vi "报文解析子VI.vi"(11 "剔除报文标识字符串":string) -> (0 "当时日期":string, 1 "速度及航向":string, 2 "经度":string, 3 "纬度":string, 4 "UTCtime":string)   [LabVIEW 2018]
panel:
  out "对地真航向":string
  out "对地速度":string
  out "ULon":string
  out "LON":string
  out "ULat":string
  out "LAT":string
  out "STATUS":u8[](array[numeric])
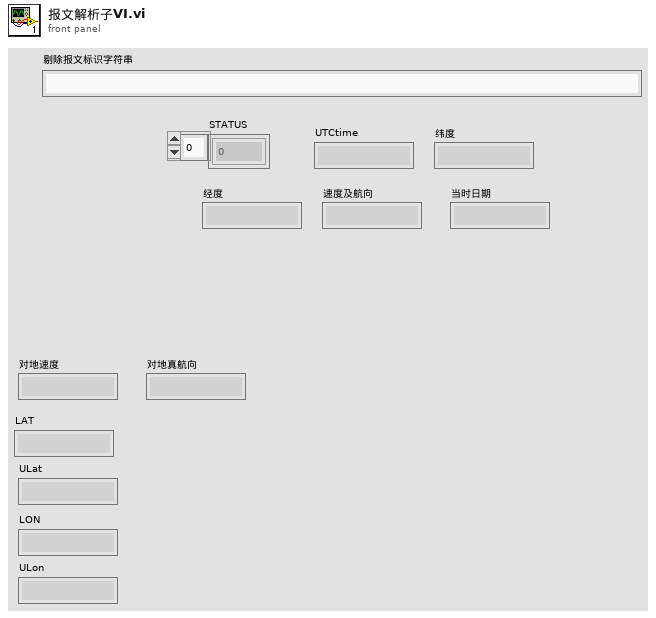
[diagram p1: front panel]
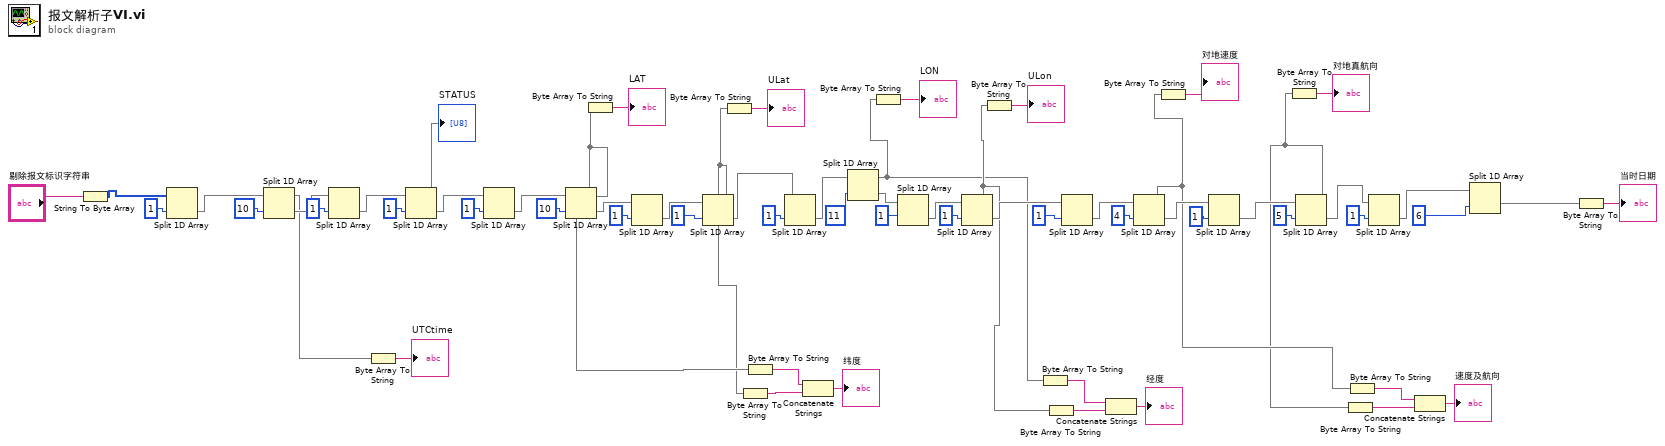
[diagram p0: block diagram]
diagram:
  n1 = String To Byte Array(string="剔除报文标识字符串") -> (unsigned byte array=w26:u8[])
  n2 = Split 1D Array(array=w26, index=1 ("索引")) -> (second subarray=w62:u8[])  [unwired: 1 out]
  n3 = Split 1D Array(array=w62, index=10 ("索引")) -> (first subarray=w25:u8[], second subarray=w60:u8[])
  n4 = Split 1D Array(array=w60, index=1 ("索引")) -> (second subarray=w58:u8[])  [unwired: 1 out]
  n5 = Byte Array To String(unsigned byte array=w25) -> (string=→"UTCtime":string)
  n6 = Split 1D Array(array=w58, index=1 ("索引")) -> (first subarray=→"STATUS":u8[], second subarray=w55:u8[])
  n7 = Split 1D Array(array=w55, index=1 ("索引")) -> (second subarray=w53:u8[])  [unwired: 1 out]
  n8 = Split 1D Array(array=w53, index=10 ("索引")) -> (first subarray=w15:u8[], second subarray=w51:u8[])
  n9 = Byte Array To String(unsigned byte array=w15) -> (string=→"LAT":string)
  n10 = Split 1D Array(array=w51, index=1 ("索引")) -> (second subarray=w49:u8[])  [unwired: 1 out]
  n11 = Split 1D Array(array=w49, index=1 ("索引")) -> (first subarray=w14:u8[], second subarray=w47:u8[])
  n12 = Byte Array To String(unsigned byte array=w14) -> (string=→"ULat":string)
  n13 = Byte Array To String(unsigned byte array=w14) -> (string=w3:string)
  n14 = Byte Array To String(unsigned byte array=w15) -> (string=w4:string)
  n15 = Split 1D Array(array=w47, index=1 ("索引")) -> (second subarray=w45:u8[])  [unwired: 1 out]
  n16 = Concatenate Strings(w4, w3) -> (→"纬度":string)
  n17 = Split 1D Array(array=w45, index=11 ("索引")) -> (first subarray=w12:u8[], second subarray=w43:u8[])
  n18 = Byte Array To String(unsigned byte array=w12) -> (string=→"LON":string)
  n19 = Split 1D Array(array=w43, index=1 ("索引")) -> (second subarray=w41:u8[])  [unwired: 1 out]
  n20 = Split 1D Array(array=w41, index=1 ("索引")) -> (first subarray=w13:u8[], second subarray=w39:u8[])
  n21 = Byte Array To String(unsigned byte array=w13) -> (string=→"ULon":string)
  n22 = Byte Array To String(unsigned byte array=w12) -> (string=w9:string)
  n23 = Byte Array To String(unsigned byte array=w13) -> (string=w8:string)
  n24 = Split 1D Array(array=w39, index=1 ("索引")) -> (second subarray=w37:u8[])  [unwired: 1 out]
  n25 = Concatenate Strings(w9, w8) -> (→"经度":string)
  n26 = Split 1D Array(array=w37, index=4 ("索引")) -> (first subarray=w11:u8[], second subarray=w35:u8[])
  n27 = Byte Array To String(unsigned byte array=w11) -> (string=→"对地速度":string)
  n28 = Split 1D Array(array=w35, index=1 ("索引")) -> (second subarray=w33:u8[])  [unwired: 1 out]
  n29 = Split 1D Array(array=w33, index=5 ("索引")) -> (first subarray=w10:u8[], second subarray=w31:u8[])
  n30 = Byte Array To String(unsigned byte array=w10) -> (string=→"对地真航向":string)
  n31 = Byte Array To String(unsigned byte array=w10) -> (string=w1:string)
  n32 = Byte Array To String(unsigned byte array=w11) -> (string=w2:string)
  n33 = Split 1D Array(array=w31, index=1 ("索引")) -> (second subarray=w29:u8[])  [unwired: 1 out]
  n34 = Concatenate Strings(w2, w1) -> (→"速度及航向":string)
  n35 = Split 1D Array(array=w29, index=6 ("索引")) -> (first subarray=w23:u8[])  [unwired: 1 out]
  n36 = Byte Array To String(unsigned byte array=w23) -> (string=→"当时日期":string)
